vi "INIT_external.vi"(8 "error in (no error)":errorcluster, 11 "UV-VIS_AVANTES in":refnum<class "UV-VIS_AVANTES.lvclass">) -> (0 "error out":errorcluster, 3 "UV-VIS_AVANTES out":refnum<class "UV-VIS_AVANTES.lvclass">)   [LabVIEW 2020]
uses:
  UV-VIS_AVANTES.lvclass
  GeneralFunctionality/GeneralFunctionality.lvclass
  Config/Config.lvclass
  C:/Dev/TRANCON/Classes/Detector/Detector.lvclass
  C:/Dev/TRANCON/Classes/GeneralFunctionality/GeneralFunctionality.lvclass
  C:/Dev/TRANCON/Classes/Detector/UV-VIS_AVANTES/UV-VIS_AVANTES.lvclass
  Detector.lvclass
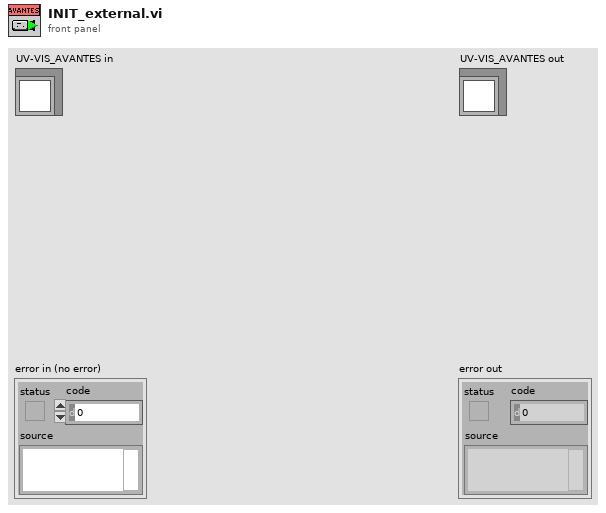
[diagram p1: front panel]
types:
  T1 = typedef "UV-VIS_AVANTES.lvclass/def_parameters.ctl" = cluster{"Len":u16, "ConfigVersion":u16, "UserFriendlyId":u8[], "DetectorType":cluster{"SensorType":u8, "NrPixels":u16, "Fit":sgl[], "NLEnable":u8, "NLCorrect":dbl[], "LowNLCounts":dbl, "HighNLCounts":dbl, "Gain":sgl[], "Reserved":sgl, "Offset":sgl[], "Extern Offset":sgl, "DefectivePixels":u16[]}, "IrradianceType":cluster{"SpectrumCalibrationType":cluster{"SmoothingType":cluster{"m_SmoothPix":u16, "SmoothModel":u8}, "CalInttime":sgl, "CalibConvers":sgl[]}, "CalibrationType":u8, "FiberDiameter":i32}, "SpectrumCalibrationType":cluster{"SmoothingType":cluster{"m_SmoothPix":u16, "SmoothModel":u8}, "CalInttime":sgl, "CalibConvers":sgl[]}, "SpectrumCorrectionType":sgl[], "StandAloneType":cluster{"StandAloneType":u8, "MeasConfigType":cluster{"StartPixel":u16, "StopPixel":u16, "IntegrationTime":sgl, "IntegrationDelay":u32, "NrAverages":u32, "DarkCorrectionType":cluster{"Enable CorDynDark":u8, "ForgetPercentage":u8}, "SmoothingType":cluster{"SmoothPix":u16, "SmoothModel":u8}, "SatDetection":u8, "TriggerType":cluster{"Trigger Mode":u8, "Trigger Source":u8, "Trigger SourceType":u8}, "ControlSettingsType":cluster{"StrobeControl":u16, "LaserDelay":u32, "LaserWidth":u32, "LaserWaveLength":sgl, "StoreToRam":u16}}, "Nmsr":i16}, "DynamicStorageType":cluster{"Nmsr":i32, "Reserved":u8[]}, "TempSensorType":sgl[], "TecControlType":cluster{"Enable":u8, "Setpoint":sgl, "Fit[NR_DAC_POL_COEF]":sgl[]}, "ProcessControlType":cluster{"AnalogLow":sgl[], "AnalogHigh":sgl[], "DigitalLow":sgl[], "DigitalHigh":sgl[]}, "EthernetSettingsType":cluster{"IpAddr":u32, "NetMask":u32, "Gateway":u32, "DhcpEnabled":u8, "TcpPort":u16, "LinkStatus":u8}, "Reserved":u8[]}
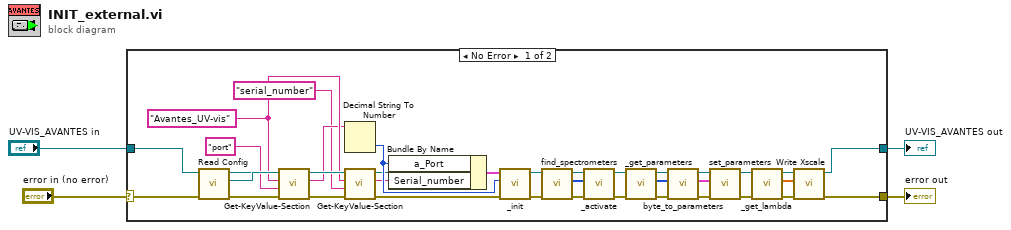
[diagram p0: block diagram]
diagram:
  n1 = case shown="No Error" "error in (no error)" {
    selector: "error in (no error)" -> [w24 w40]
    tunnel: [w6 w41] -> w3
    tunnel: "UV-VIS_AVANTES in" -> [w34 w41]
    tunnel: [w5 w40] -> w1
    frame No Error {
      w30 = "Avantes_UV-vis" ("Section")
      n2 = call "Read Config.vi"("error in (no error)"=w24, "GeneralFunctionality en entrée"=w34) -> ("error out"=w33:errorcluster, "Config.lvclass"=w35:refnum<class "Config.lvclass">, "GeneralFunctionality en sortie"=w23:refnum<class "UV-VIS_AVANTES.lvclass">)  [unwired: 7 in]
      n3 = call-dynamic "Get-KeyValue-Section.vi"("error in (no error)"=w33, "Key"="port", "Section"=w30, "Config in"=w35) -> ("error out"=w32:errorcluster, "Value"=w28:string, "Config out"=w31:refnum<class "Config.lvclass">)  [unwired: 5 in]
      n4 = Decimal String To Number(string=w28) -> (number=w27:i32)  [unwired: 2 in, 1 out]
      n5 = call-dynamic "Get-KeyValue-Section.vi"("error in (no error)"=w32, "Key"="serial_number", "Section"=w30, "Config in"=w31) -> ("error out"=w21:errorcluster, "Value"=w25:string)  [unwired: 5 in, 1 out]
      n6 = Bundle By Name(cluster=w23, "a_Port"=w27, "Serial_number"=w25) -> (w22:cluster{})
      n7 = call "_init.vi"("error in (no error)"=w21, "a_Port"=w27, "UV-VIS_AVANTES in"=w22) -> ("error out"=w37:errorcluster, "UV-VIS_AVANTES out"=w38:refnum<class "UV-VIS_AVANTES.lvclass">)  [unwired: 6 in, 1 out]
      n8 = call "find_spectrometers.vi"("error in (no error)"=w37, "UV-VIS_AVANTES in"=w38) -> ("error out"=w36:errorcluster, "List Output"=w20:u8[], "UV-VIS_AVANTES out"=w39:refnum<class "UV-VIS_AVANTES.lvclass">)  [unwired: 7 in]
      n9 = call "_activate.vi"("error in (no error)"=w36, "a_pDeviceId IN"=w20, "UV-VIS_AVANTES in"=w39) -> ("error out"=w12:errorcluster, "UV-VIS_AVANTES out"=w13:refnum<class "UV-VIS_AVANTES.lvclass">)  [unwired: 7 in]
      n10 = call "_get_parameters.vi"("error in (no error)"=w12, "UV-VIS_AVANTES in"=w13) -> ("error out"=w19:errorcluster, "DeviceParam"=w18:u8[], "UV-VIS_AVANTES out"=w14:refnum<class "UV-VIS_AVANTES.lvclass">)  [unwired: 7 in]
      n11 = call "byte_to_parameters.vi"("error in (no error)"=w19, "DeviceParam"=w18, "UV-VIS_AVANTES in"=w14) -> ("error out"=w15:errorcluster, "parameters cluster"=w17:T1, "UV-VIS_AVANTES out"=w16:refnum<class "UV-VIS_AVANTES.lvclass">)  [unwired: 6 in]
      n12 = call "set_parameters.vi"("error in (no error)"=w15, "AVS_parameters"=w17, "UV-VIS_AVANTES in"=w16) -> ("error out"=w10:errorcluster, "UV-VIS_AVANTES out"=w9:refnum<class "UV-VIS_AVANTES.lvclass">)  [unwired: 7 in]
      n13 = call "_get_lambda.vi"("error in (no error)"=w10, "UV-VIS_AVANTES in"=w9) -> ("error out"=w7:errorcluster, "a_pWaveLength"=w11:dbl[], "UV-VIS_AVANTES out"=w8:refnum<class "UV-VIS_AVANTES.lvclass">)  [unwired: 7 in]
      n14 = call "Write Xscale.vi"("error in (no error)"=w7, "Xscale"=w11, "Detector en entrée"=w8) -> ("error out"=w5:errorcluster, "Detector en sortie"=w6:refnum<class "UV-VIS_AVANTES.lvclass">)  [unwired: 7 in]
    }
    frame Error {
    }
  }
  "error out" <- w1
  "UV-VIS_AVANTES out" <- w3
